vi "Module Data - Append Newly Handled Error.vi"(2 "Index of the newly reported error in the OSI data structure":i32, 3 "Newly Reported Error":T9, 4 "Module Data in":T3) -> (0 "Error to be logged to file":T1, 1 "Module Data out (Error appended)":T3)   [LabVIEW 2023, in "Error Manager.lvlib"]
doc: "Blank VI with error handling."
uses:
  Error Manager.lvlib
  Module Data (cluster).ctl
  GUI Object References (cluster).ctl
  Handled Error (cluster).ctl
  Read-Unread Status (enum).ctl
  Display Order (enum).ctl
  Error in current one-second interval (cluster).ctl
  Reported Error (cluster).ctl
  Public API VIs/Show Error Window Instruction (enum).ctl
  Error Log/Error to be logged (cluster).ctl
  Error Log/Error Type (enum).ctl
  Error Log/Error Log.lvclass
panel:
  out "Total no. of errors handled so far":i32
  # "Input\nInputs to the VI"
  # "Development\nControls or indicators that are useful for development or testing, but which are not outputs of the VI."
  # "Output\nOutputs of the VI"
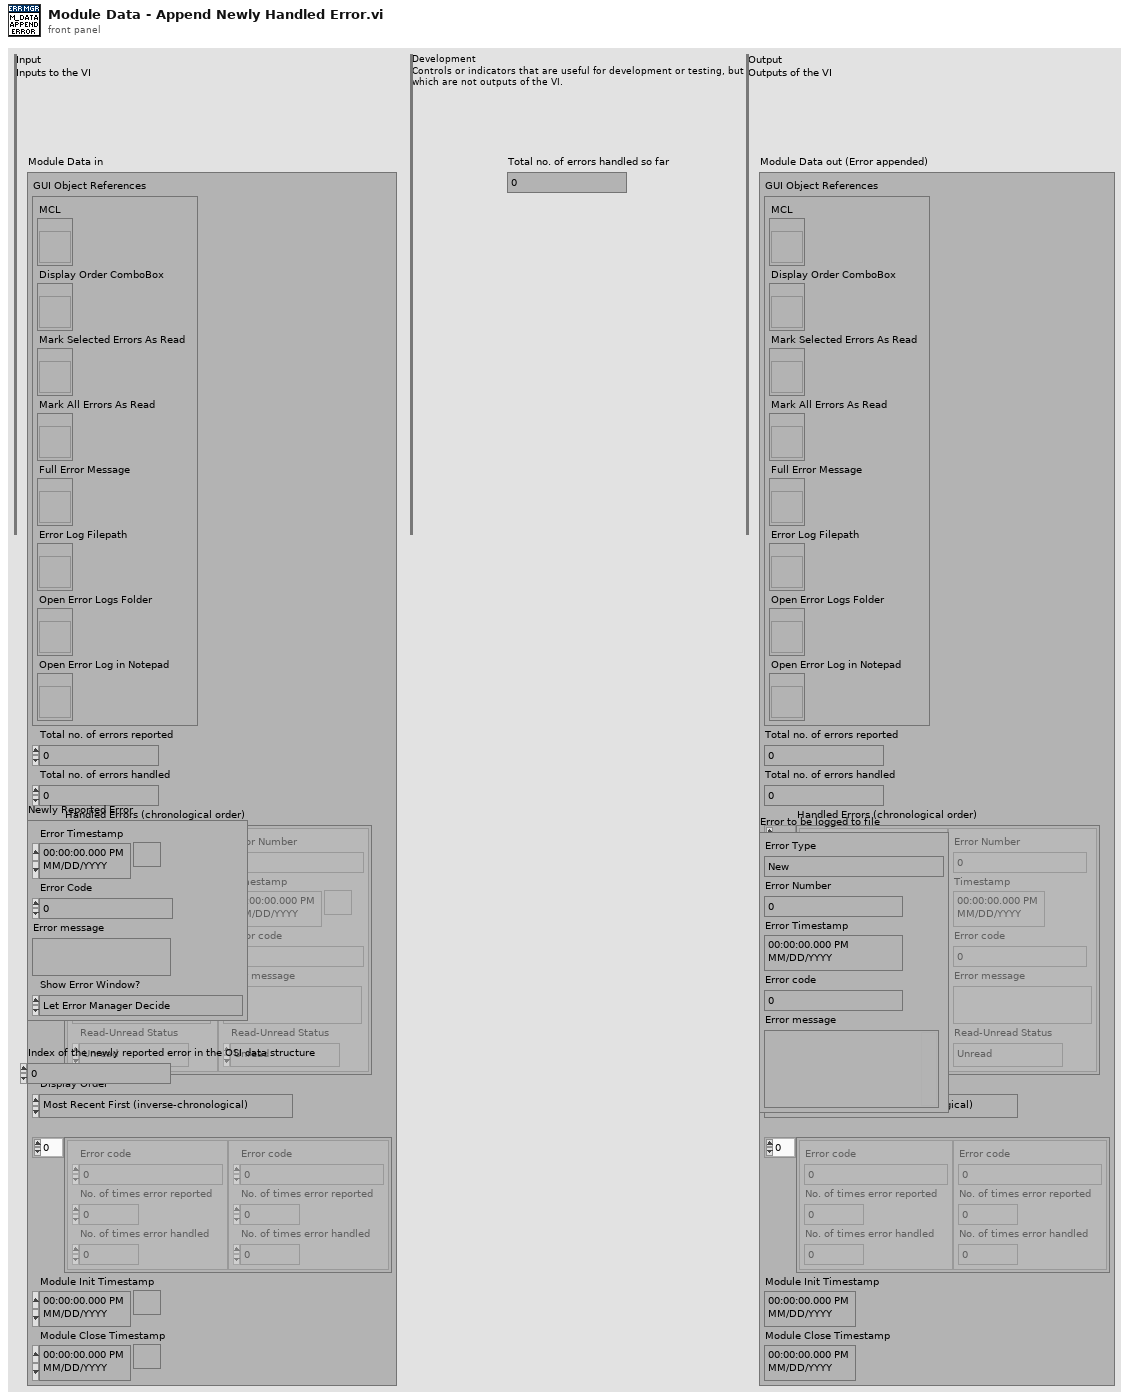
[diagram p1: front panel]
types:
  T1 = typedef "Error Manager.lvlib/Error Log.lvclass/Error to be logged (cluster).ctl" = cluster{"Error Type":T2, "Error Number":i32, "Error Timestamp":timestamp, "Error code":i32, "Error message":string}
  T2 = typedef "Error Manager.lvlib/Error Log.lvclass/Error Type (enum).ctl" = enum16{"New", "Identical to last logged error"}
  T3 = typedef "Error Manager.lvlib/Module Data (cluster).ctl" = cluster{"GUI Object References":T4, "Total no. of errors reported":i32, "Total no. of errors handled":i32, "Handled Errors (chronological order)":T5[], "Display Order":T7, "Errors in current one-second interval":T8[], "Module Init Timestamp":timestamp, "Module Close Timestamp":timestamp}
  T4 = typedef "Error Manager.lvlib/GUI Object References (cluster).ctl" = cluster{"MCL":refnum<vi>, "Display Order ComboBox":refnum<vi>, "Mark Selected Errors As Read":refnum<vi>, "Mark All Errors As Read":refnum<vi>, "Full Error Message":refnum<vi>, "Error Log Filepath":refnum<vi>, "Open Error Logs Folder":refnum<vi>, "Open Error Log in Notepad":refnum<vi>}
  T5 = typedef "Error Manager.lvlib/Handled Error (cluster).ctl" = cluster{"Error Number":i32, "Timestamp":timestamp, "Error code":i32, "Error message":string, "Read-Unread Status":T6}
  T6 = typedef "Error Manager.lvlib/Read-Unread Status (enum).ctl" = enum16{"Unread", "Read"}
  T7 = typedef "Error Manager.lvlib/Display Order (enum).ctl" = enum16{"Most Recent First (inverse-chronological)", "Oldest First (chronological)"}
  T8 = typedef "Error Manager.lvlib/Error in current one-second interval (cluster).ctl" = cluster{"Error code":i32, "No. of times error reported":u32, "No. of times error handled":u32}
  T9 = typedef "Error Manager.lvlib/Reported Error (cluster).ctl" = cluster{"Error Timestamp":timestamp, "Error Code":i32, "Error message":string, "Show Error Window?":T10}
  T10 = typedef "Error Manager.lvlib/Show Error Window Instruction (enum).ctl" = enum16{"Let Error Manager Decide", "Show", "Do Not Show"}
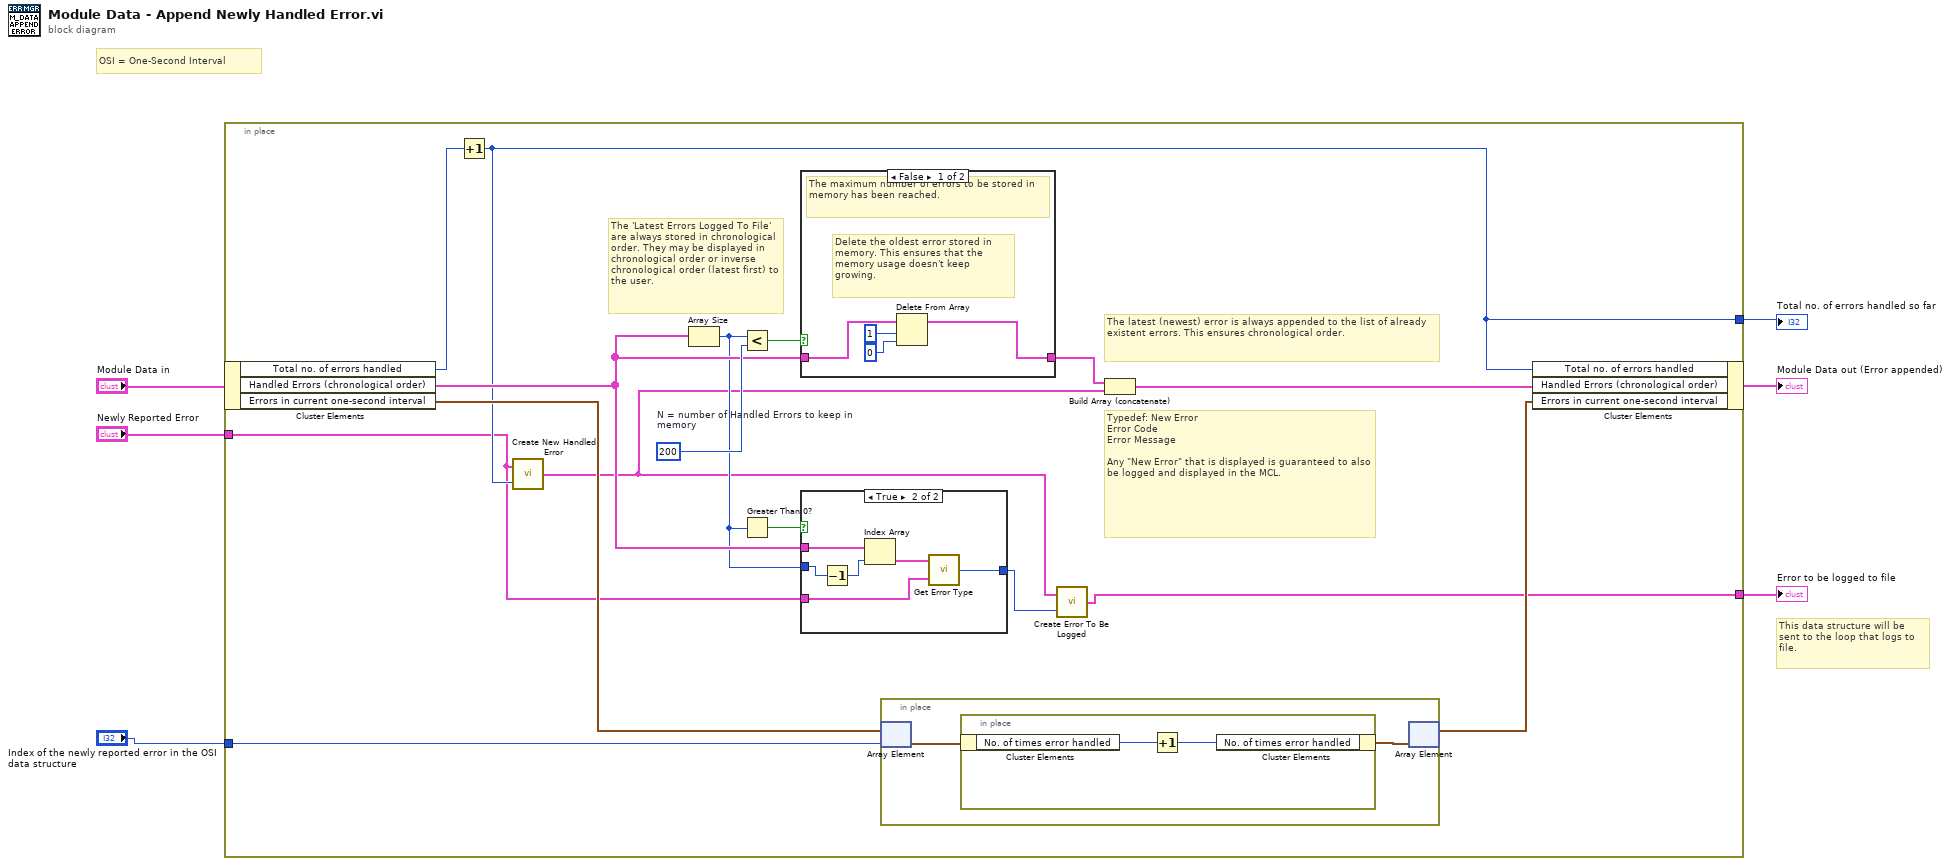
[diagram p0: block diagram]
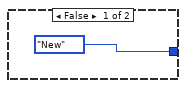
[diagram p2: hidden frame]
diagram:
  # "This data structure will be sent to the loop that logs to file."
  # "OSI = One-Second Interval"
  n1 = in-place {
    in-place-border: "Newly Reported Error" -> [w10]
    in-place-border: [w11] -> w2
    in-place-border: "Index of the newly reported error in the OSI data structure" -> [w20]
    in-place-border: [w8] -> w1
    w18 = 200  # N = number of Handled Errors to keep in memory
    # "Typedef: New Error\nError Code\nError Message\n\nAny \"New Error\" that is displayed is guaranteed to also be logged and displayed in the MCL."
    # "The 'Latest Errors Logged To File' are always stored in chronological order. They may be displayed in chronological order or inverse chronological order (latest first) to the user."
    # "The latest (newest) error is always appended to the list of already existent errors. This ensures chronological order."
    n2 = in-place-cluster #1("Module Data in") -> ("Total no. of errors handled"=w15:i32, "Handled Errors (chronological order)"=w13:T5[], "Errors in current one-second interval"=w21:T8[])
    n3 = Increment(x=w15) -> (x+1=w11:i32)
    n4 = call "Create New Handled Error.vi"("Error Number"=w11, "Reported Error"=w10) -> ("Handled Error"=w7:T5)
    n5 = Array Size(array=w13) -> (size(s)=w12:i32)
    n6 = Less?(x=w12, y=w18) -> (x < y?=w17:bool)
    n7 = Greater Than 0?(x=w12) -> (x > 0?=w14:bool)
    n8 = case shown="False" w17 {
      tunnel: w13 -> [w33 w34]
      tunnel: [w30 w34] -> w16
      frame False {
        # "Delete the oldest error stored in memory. This ensures that the memory usage doesn't keep growing."
        # "The maximum number of errors to be stored in memory has been reached."
        n9 = Delete From Array(array=w33, length=1, index=0) -> (array with subset deleted=w30:T5[])  [unwired: 1 out]
      }
      frame True {
      }
    }
    n10 = case shown="True" w14 {
      tunnel: [Error_Type_(enum)."New" ("Error Type") w24] -> w9
      tunnel: w13 -> [_ w29]
      tunnel: w12 -> [_ w28]
      tunnel: w10 -> [_ w25]
      frame False {
      }
      frame True {
        n11 = Decrement(x=w28) -> (x-1=w27:i32)
        n12 = Index Array(array=w29, index=w27) -> (element=w26:T5)
        n13 = call "Get Error Type.vi"("Newly Reported Error"=w25, "Last (latest) Handled Error"=w26) -> ("Error Type"=w24:T2)
      }
    }
    n14 = in-place {
      n15 = in-place-array #2(w21, w20) -> (w36:T8)
      n16 = in-place {
        n17 = in-place-cluster #3(w36) -> ("No. of times error handled"=w38:u32)
        n18 = Increment(x=w38) -> (x+1=w37:u32)
        n19 = in-place-cluster #3("No. of times error handled"=w37) -> (w35:T8)
      }
      n20 = in-place-array #2(w35) -> (w19:T8[])  [unwired: 1 out]
    }
    n21 = call "Create Error To Be Logged.vi"("Error Type"=w9, "Handled Error"=w7) -> ("Error to be logged to file"=w8:T1)
    n22 = Build Array (concatenate)(w16, w7) -> (w22:T5[])
    n23 = in-place-cluster #1("Total no. of errors handled"=w11, "Handled Errors (chronological order)"=w22, "Errors in current one-second interval"=w19) -> (→"Module Data out (Error appended)":T3)
  }
  "Total no. of errors handled so far" <- w2
  "Error to be logged to file" <- w1
